vi "PostScanUpdate.vi"(8 "error in (no error)":errorcluster caption="entrée d'erreur (pas d'erreur)", 10 "PostScanString":string, 11 "Interface en entrée":refnum<class "Interface.lvclass"> caption="DNL_LabVIEW Object in") -> (0 "error out":errorcluster caption="sortie d'erreur", 3 "Interface en sortie":refnum<class "Interface.lvclass"> caption="DNL_LabVIEW Object out")   [LabVIEW 2019, in "Interface.lvclass"]
uses:
  Interface.lvclass
  Interface.lvclass/Interface.ctl
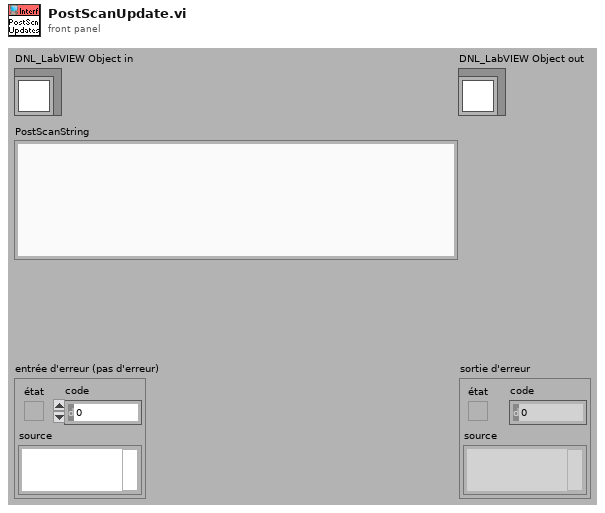
[diagram p1: front panel]
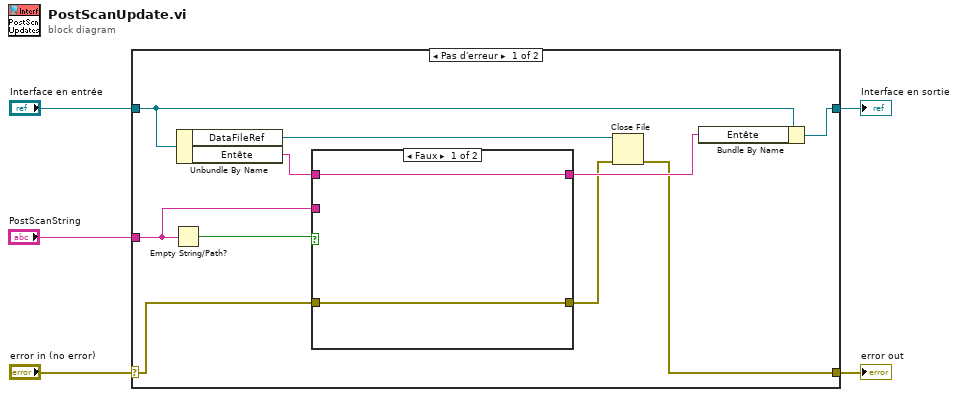
[diagram p0: block diagram]
diagram:
  n1 = case shown="Pas d'erreur" "error in (no error)" {
    selector: "error in (no error)" -> [w7 w21]
    tunnel: [w9 w21] -> w4
    tunnel: [w14 w20] -> w2
    tunnel: "Interface en entrée" -> [w15 w20]
    tunnel: "PostScanString" -> [w10 _]
    frame No Error {
      n2 = Empty String/Path?(string/path=w10) -> (empty?=w13:bool)
      n3 = Unbundle By Name(w15) -> ("DataFileRef"=w8:refnum<file>, "Entête"=w11:string)
      n4 = case shown="Faux" w13 {
        tunnel: [w17 w19] -> w12
        tunnel: w11 -> [w17 w19]
        tunnel: w10 -> [_ _]
        tunnel: w7 -> [w16 w18]
        tunnel: [w16 w18] -> w6
        frame False {
        }
        frame True {
        }
      }
      n5 = Close File(refnum=w8, error in=w6) -> (error out=w9:errorcluster)  [unwired: 1 out]
      n6 = Bundle By Name(cluster=w15, "Entête"=w12) -> (w14:refnum<class "Interface.lvclass">)
    }
    frame Error {
    }
  }
  "error out" <- w4
  "Interface en sortie" <- w2
